vi "Open All Relays.vi"(8 "error in":errorcluster, 11 "SwitchMatrix in":refnum<class "SwitchMatrix.lvclass">) -> (0 "error out":errorcluster, 3 "SwitchMatrix out":refnum<class "SwitchMatrix.lvclass">)   [LabVIEW 2019, in "SwitchMatrix.lvlib" / "SwitchMatrix.lvclass"]
doc: "Open all relays is a static implementation because the state information in memory must be updated before opening the relays. This allows the end user to be aware of the switch state without requiring a query to the instrument."
uses:
  Library/SwitchMatrix.lvclass
  C:/Users/Public/Documents/Development/builds/Instruments/Instruments.lvlibp/Library/Instruments.lvclass
  Library/SwitchMatrix.lvclass/SwitchMatrix.ctl
  builds/Instruments/Instruments.lvlibp/Private/Polymorphic/Special/Event from String.vi
  builds/Instruments/Instruments.lvlibp/Accessors/Command with Logging.vi
  builds/Instruments/Instruments.lvlibp/Library/Instruments.lvclass
  builds/Instruments/Instruments.lvlibp
  builds/Engine/Engine.lvlibp/Project/Engine.lvclass
  C:/Users/Public/Documents/Development/builds/Engine/Engine.lvlibp/Project/Engine.lvclass
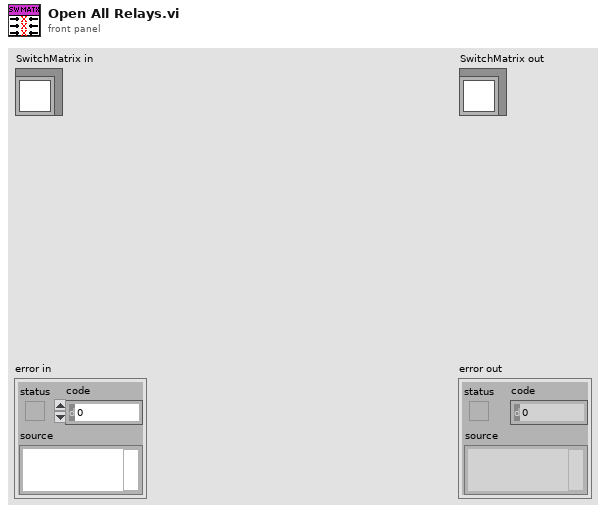
[diagram p1: front panel]
types:
  T1 = cluster{"Timestamp":timestamp, "Description":string, "Data":string}
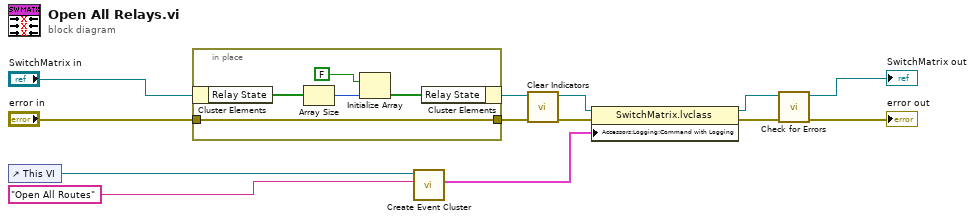
[diagram p0: block diagram]
diagram:
  n1 = control-ref of="This VI"() -> (w7:refnum<vi>)
  n2 = in-place {
    in-place-border: "error in" -> [w18]
    in-place-border: [w18] -> w10
    n3 = in-place-cluster #1("SwitchMatrix in") -> ("Relay State"=w17:bool[])
    n4 = Array Size(array=w17) -> (size(s)=w16:i32)
    n5 = Initialize Array(FALSE, w16) -> (w14:bool[])
    n6 = in-place-cluster #1("Relay State"=w14) -> (w11:refnum<class "SwitchMatrix.lvclass">)
  }
  n7 = call-poly "Create Event Cluster.vi"("Value"="Open All Routes", "VI Refnum"=w7) -> ("Event Data"=w6:T1)  [unwired: 9 in]
  n8 = call "Clear Indicators.vi"("error in"=w10, "SwitchMatrix in"=w11) -> ("error out"=w8:errorcluster, "SwitchMatrix out"=w9:refnum<class "SwitchMatrix.lvclass">)  [unwired: 8 in]
  n9 = property class="SwitchMatrix.lvclass"(reference=w9, error in=w8, "Accessors:Logging:Command with Logging"=w6) -> (reference out=w3:refnum<class "SwitchMatrix.lvclass">, error out=w4:errorcluster)
  n10 = call "Check for Errors.vi"("error in"=w4, "Engine in"=w3) -> ("error out"=→"error out":errorcluster, "Engine out"=→"SwitchMatrix out":refnum<class "SwitchMatrix.lvclass">)  [unwired: 8 in]
